vi "epxMAUpdate.vi"(6 "inputValid":bool, 8 "expFactor":i16=-8, 10 "update":i16, 11 "carryIn":fxp<+/-,22,16>) -> (3 "carryOut":fxp<+/-,22,16>, 4 "outputValid":bool)   [LabVIEW 2016]
uses:
  <vilib>/rvi/FXPMathLib/FxpSub/XNode/nifxpmath_Sub.xnode
  <vilib>/rvi/FXPMathLib/FxpAdd/XNode/nifxpmath_Add.xnode
  <vilib>/rvi/FXPMathLib/sim/FxpSim.dll
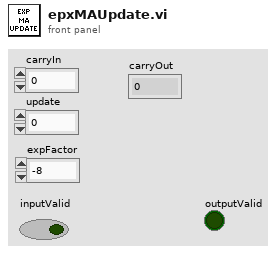
[diagram p1: front panel]
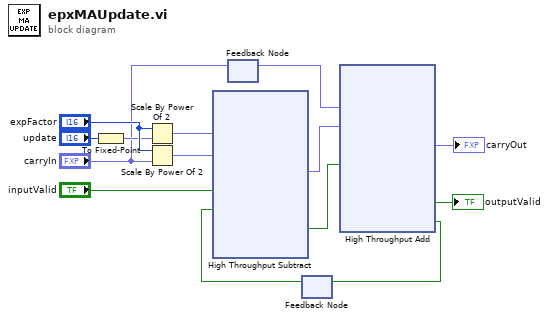
[diagram p0: block diagram]
diagram:
  n1 = To Fixed-Point(number="update") -> (fixed-point=w9:fxp<+/-,22,16>)  [unwired: 1 in]
  n2 = Scale By Power Of 2(n="expFactor", x=w9) -> (x*2^n=w7:fxp<+/-,22,16>)
  n3 = Scale By Power Of 2(n="expFactor", x="carryIn") -> (x*2^n=w6:fxp<+/-,22,16>)
  n4 = feedback-in #1("carryIn") -> ()
  n5 = feedback #1() -> (w1:fxp<+/-,22,16>)  [unwired: 1 in]
  n6 = feedback #2() -> (w10:bool)  [unwired: 1 in]
  n7 = xnode "High Throughput Subtract"("x"=w7, "y"=w6, "input valid"="inputValid", "ready for output (T)"=w10) -> ("x-y"=w5:fxp<+/-,22,16>, "output valid"=w12:bool)  [unwired: 1 out]
  n8 = xnode ("High Throughput Add")("x"=w1, "y"=w5, "input valid"=w12) -> ("x+y"=→"carryOut":fxp<+/-,22,16>, "output valid"=→"outputValid":bool, "ready for input"=w11:bool)  [unwired: 1 in]
  n9 = feedback-in #2(w11) -> ()
